vi "InitializeCore.vi"(8 "error in (no error)":errorcluster, 10 "Micron Args":T1, 11 "MicronServer in":refnum<class "GRPCService.lvclass">) -> (0 "error out":errorcluster, 2 "MessageUserEvent":refnum<user-event>, 3 "MicronServer out":refnum<class "GRPCService.lvclass">)   [LabVIEW 2019, in "MicronGRPCServer.lvlib" / "GRPCService.lvclass"]
uses:
  GRPCService.lvclass
  Base/Server/Message/MessageBase.lvclass
  Base/Server/Service/Typedefs/MicronArgs.ctl
  MicronCLI/Typedefs/ServiceDetails.ctl
  GRPCService.lvclass/GRPCService.ctl
  MicronCLI/MicronCLI.lvclass
  Generated/MicronGRPCGeneratedServer/MicronGRPCGeneratedServer.lvlib
  Base/Server/Service/ServiceBase.lvclass
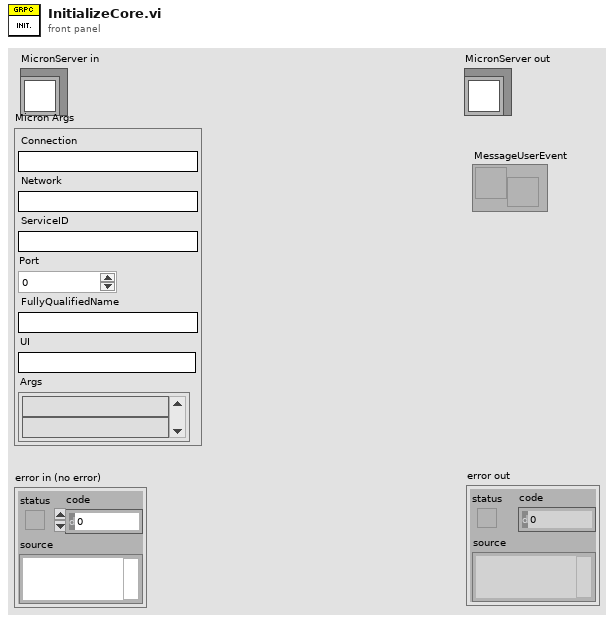
[diagram p1: front panel]
types:
  T1 = typedef "MicronServer.lvlib/ServiceBase.lvclass/MicronArgs.ctl" = cluster{"Connection":string, "Network":string, "ServiceID":string, "Port":i32, "FullyQualifiedName":string, "UI":string, "Args":string[]}
  T2 = typedef "MicronCLI.lvclass/ServiceDetails.ctl" = cluster{"Network":string, "ServiceID":string}
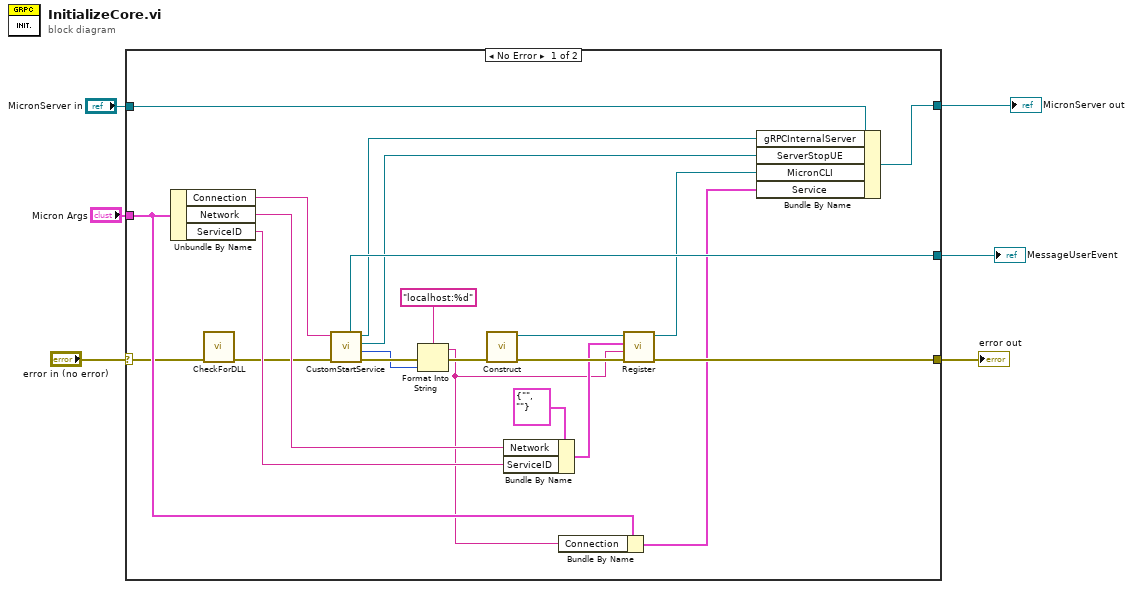
[diagram p0: block diagram]
diagram:
  n1 = case shown="No Error" "error in (no error)" {
    selector: "error in (no error)" -> [w7 w30]
    tunnel: [w28 _] -> w5
    tunnel: "MicronServer in" -> [w27 w31]
    tunnel: [w26 w31] -> w3
    tunnel: [w19 w30] -> w2
    tunnel: "Micron Args" -> [w11 _]
    frame No Error {
      n2 = Unbundle By Name(w11) -> ("Connection"=w17:string, "Network"=w15:string, "ServiceID"=w14:string)
      n3 = call "CheckForDLL.vi"("error in"=w7) -> ("error out"=w8:errorcluster)  [unwired: 10 in]
      n4 = call "CustomStartService.vi"("error in"=w8, "Server Address"=w17) -> ("error out"=w29:errorcluster, "Listening Port"=w21:i32, "Server Stop"=w24:refnum<user-event>, "gRPC Server out"=w25:refnum<class "Servicer.lvclass">, "MicronUE"=w28:refnum<user-event>)  [unwired: 5 in]
      n5 = Format Into String(format string="localhost:%d", error in=w29, w21) -> (resulting string=w9:string, error out=w22:errorcluster)  [unwired: 1 in]
      n6 = call "Construct.vi"("error in (no error)"=w22) -> ("error out"=w23:errorcluster, "MicronCLI out"=w18:refnum<class "MicronCLI.lvclass">)  [unwired: 9 in]
      n7 = Bundle By Name(cluster=T2 {"Network"="", "ServiceID"=""} ("Service"), "Network"=w15, "ServiceID"=w14) -> (w13:T2)
      n8 = Bundle By Name(cluster=w11, "Connection"=w9) -> (w10:T1)
      n9 = call-dynamic "Register.vi"("error in (no error)"=w23, "ConnectionString"=w9, "Service"=w13, "MicronCLI in"=w18) -> ("error out"=w19:errorcluster, "MicronCLI out"=w12:refnum<class "MicronCLI.lvclass">)  [unwired: 6 in]
      n10 = Bundle By Name(cluster=w27, "gRPCInternalServer"=w25, "ServerStopUE"=w24, "MicronCLI"=w12, "Service"=w10) -> (w26:refnum<class "GRPCService.lvclass">)
    }
    frame Error {
    }
  }
  "error out" <- w2
  "MicronServer out" <- w3
  "MessageUserEvent" <- w5
